vi "Write ID.vi"(8 "error in (no error)":errorcluster, 10 "ID":u32, 11 "Socket in":refnum<class "Socket.lvclass">) -> (0 "error out":errorcluster, 3 "Socket out":refnum<class "Socket.lvclass">)   [LabVIEW 2018, in "Socket.lvclass"]
uses:
  Socket.lvclass
  Socket.lvclass/Socket.ctl
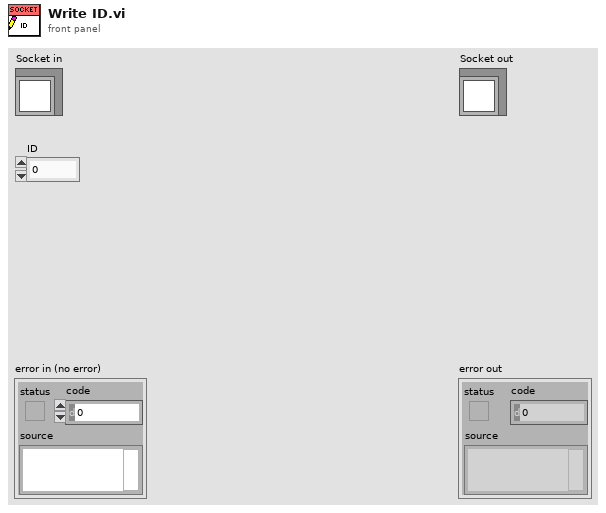
[diagram p1: front panel]
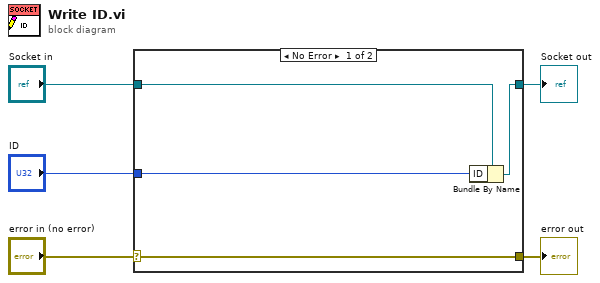
[diagram p0: block diagram]
diagram:
  n1 = case shown="No Error" "error in (no error)" {
    selector: "error in (no error)" -> [w9 w10]
    tunnel: [w9 w10] -> w4
    tunnel: [w7 w11] -> w2
    tunnel: "Socket in" -> [w8 w11]
    tunnel: "ID" -> [w6 _]
    frame No Error {
      n2 = Bundle By Name(cluster=w8, "ID"=w6) -> (w7:refnum<class "Socket.lvclass">)
    }
    frame Error {
    }
  }
  "error out" <- w4
  "Socket out" <- w2
